vi "FaultGetValue.vi"(9 "Channel":string) -> (0 "error out":errorcluster, 1 "Channel out":string, 2 "Faulted":bool, 3 "Fault Value":dbl)   [LabVIEW 2015, in "ni-veristand-steps-runtime-lib.lvlib"]
uses:
  ni-veristand-steps-runtime-lib.lvlib
  <vilib>/NI Veristand/Execution/ChannelFaultManager/NI_VS ChannelFault ExecutionAPI.lvlib
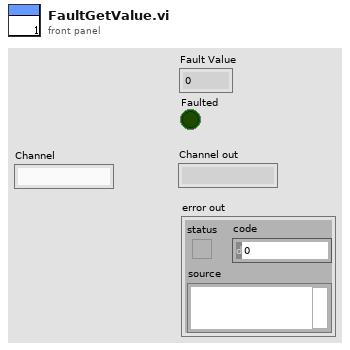
[diagram p1: front panel]
types:
  T1 = typedef "ni-veristand-steps-runtime-lib.lvlib/VeriStand dotNet References.ctl" = cluster{"Project Ref":refnum<k24>, "Workspace Manager Ref":refnum<k24>, "Model Manager Ref":refnum<k24>, "Channel Fault Manager Ref":refnum<k24>}
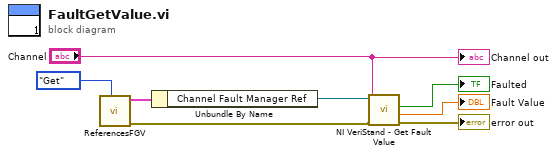
[diagram p0: block diagram]
diagram:
  n1 = call "ReferencesFGV.vi"("Get/Set"=enum16{"Get", "Set"}."Get") -> ("error out"=w2:errorcluster, "VeriStand dotNET Refs out"=w4:T1)  [unwired: 9 in]
  n2 = Unbundle By Name(w4) -> ("Channel Fault Manager Ref"=w1:refnum<k24>)
  n3 = call <vilib>:"NI VeriStand - Get Fault Value.vi"("error in (no error)"=w2, "Channel"="Channel", "ChannelFault in"=w1) -> ("error out"=→"error out":errorcluster, "Fault Value"=→"Fault Value":dbl, "Faulted"=→"Faulted":bool)  [unwired: 5 in, 1 out]
  "Channel out" <- "Channel"
